vi "Commit DAQ Tags.vi"(8 "error in (no error)":errorcluster, 11 "DAQ State in":T1) -> (0 "error out":errorcluster, 3 "DAQ State out":T1)   [LabVIEW 2018, in "DAQ.lvlib"]
uses:
  DAQ.lvlib
  Acquisition/Hardware Configuration.ctl
  Acquisition/Task Cluster.ctl
  Tag VIs/Tag FGV Operation Enum.ctl
  Shared Variables/Dynamic Shared Variables.lvlib
  <resource>/objmgr/daqmx.rc
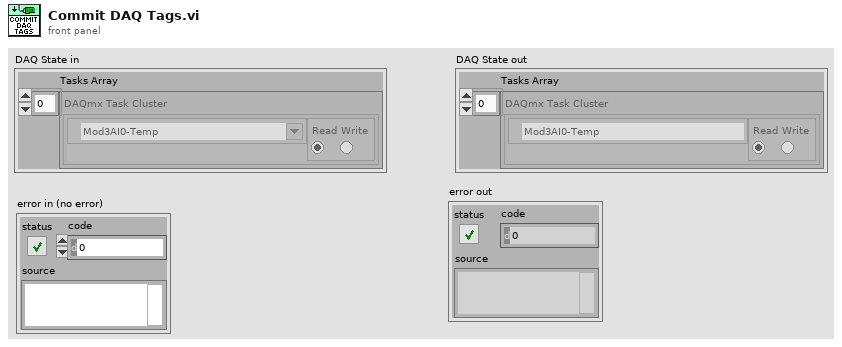
[diagram p1: front panel]
types:
  T1 = typedef "DAQ.lvlib/Hardware Configuration.ctl" = cluster{"Tasks Array":T2[]}
  T2 = typedef "Task Cluster.ctl" = cluster{"DAQmx Task":refnum<k21>, "Read-Write Radio":enum32{"Read", "Write"}}
  T3 = typedef "Tag FGV Operation Enum.ctl" = enum16{"Init", "Set Notification Queue", "Create Tag", "Commit", "Write Tag (Numeric)", "Write Tag (Boolean)", "Read All Tags", "Read One Tag", "Delete Tag Category", "Set Alarm Parameters (Numeric)", "Set Alarm Parameters (Boolean)", "Enable All Alarms", "Disable All Alarms", "Delete All Tags", "Read Alarms", "Ack Alarm", "Read Alarm Parameters (Numeric)", "Read Alarm Parameters (Boolean)"}
  T4 = cluster{"enable? (F)":bool, "name":string, "alarm on":bool, "priority":u32, "ack type":enum16{"Auto", "User", "None", "Each Occurrence"}, "area":string, "description":string, "log? (T)":bool}
  T5 = enum16{"Auto", "User", "None", "Each Occurrence"}
  T6 = enum32{"u32BitField", "bool", "double", "string", "int8", "uint8", "int16", "uint16", "int32", "uint32", "int64", "uint64", "single", "double waveform", "int16 waveform", "array of boolean", "array of int8", "array of uint8", "array of int16", "array of uint16", "array of int32", "array of uint32", "array of int64", "array of uint64", "array of single", "array of double", "array of double waveform", "array of int16 waveform", "array of string", "variant", "timestamp", "fixed point", "custom"}
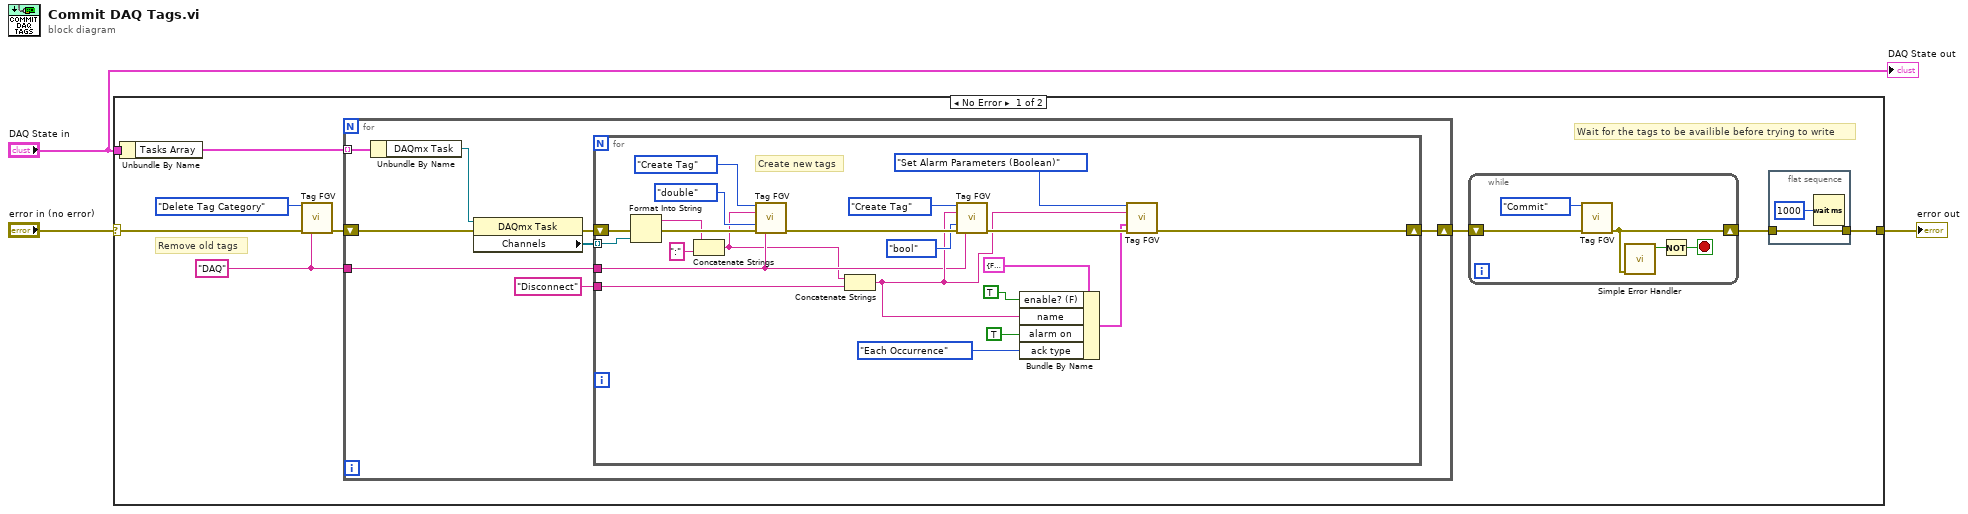
[diagram p0: block diagram]
diagram:
  n1 = case shown="No Error" "error in (no error)" {
    selector: "error in (no error)" -> [w9 w50]
    tunnel: "DAQ State in" -> [w11 _]
    tunnel: [w4 w50] -> w1
    frame No Error {
      w7 = "DAQ" ("Tag Category")
      # "Wait for the tags to be availible before trying to write"
      # "Remove old tags"
      n2 = Unbundle By Name(w11) -> ("Tasks Array"=w12:T2[])
      n3 = call "Tag FGV.vi"("Operation"=Tag_FGV_Operation_Enum."Delete Tag Category", "error in (no error)"=w9, "Tag Category"=w7) -> ("error out"=w8:errorcluster)  [unwired: 5 in, 7 out]
      n4 = for {
        tunnel: w12 -> [w27] mode=indexing
        shift-right: [w22] -> w6
        shift-left: w8 -> [w26]
        tunnel: w7 -> [w23]
        n5 = Unbundle By Name(w27) -> ("DAQmx Task"=w25:refnum<k21>)
        n6 = property class="DAQmx Task"(reference=w25, error in=w26) -> (error out=w21:errorcluster, "Channels"=w24:refnum<k21>[])  [unwired: 1 out]
        n7 = for {
          tunnel: w24 -> [w48] mode=indexing
          shift-right: [w39] -> w22
          shift-left: w21 -> [w47]
          tunnel: w23 -> [w31]
          tunnel: "Disconnect" ("string") -> [w32]
          # "Create new tags"
          n8 = Format Into String(error in=w47, w48) -> (resulting string=w30:string, error out=w49:errorcluster)  [unwired: 2 in]
          n9 = Concatenate Strings(w30, ":" ("string")) -> (w28:string)
          n10 = call "Tag FGV.vi"("Operation"=Tag_FGV_Operation_Enum."Create Tag", "Tag Name"=w28, "Data"=T6."double" ("data type"), "error in (no error)"=w49, "Tag Category"=w31) -> ("error out"=w44:errorcluster)  [unwired: 3 in, 7 out]
          n11 = Concatenate Strings(w28, w32) -> (w36:string)
          n12 = call "Tag FGV.vi"("Operation"=Tag_FGV_Operation_Enum."Create Tag", "Tag Name"=w36, "Data"=T6."bool" ("data type"), "error in (no error)"=w44, "Tag Category"=w31) -> ("error out"=w40:errorcluster)  [unwired: 3 in, 7 out]
          n13 = Bundle By Name(cluster=T4 {"enable? (F)"=FALSE, "name"="Boolean", "alarm on"=TRUE, "priority"=1, "ack type"=enum."Auto", "area"="", "description"="", "log? (T)"=TRUE} ("Boolean alarm settings"), "enable? (F)"=TRUE, "name"=w36, "alarm on"=TRUE, "ack type"=T5."Each Occurrence") -> (w33:T4)
          n14 = call "Tag FGV.vi"("Operation"=Tag_FGV_Operation_Enum."Set Alarm Parameters (Boolean)", "Tag Name"=w36, "Data"=w33, "error in (no error)"=w40) -> ("error out"=w39:errorcluster)  [unwired: 4 in, 7 out]
        }
      }
      n15 = while {
        shift-right: [w17] -> w5
        shift-left: w6 -> [w18]
        stop <- w15 stop-if-true
        n16 = call "Tag FGV.vi"("Operation"=Tag_FGV_Operation_Enum."Commit", "error in (no error)"=w18) -> ("error out"=w17:errorcluster)  [unwired: 6 in, 7 out]
        n17 = call <vilib>:"Simple Error Handler.vi"("error in (no error)"=w17) -> ("error?"=w16:bool)  [unwired: 4 in, 4 out]
        n18 = Not(x=w16) -> (.not. x?=w15:bool)
      }
      n19 = flat-sequence {
        tunnel: [w13] -> w4
        tunnel: w5 -> [w13]
        frame #0 {
          n20 = Wait (ms)(milliseconds to wait=u32 1000) -> ()  [unwired: 1 out]
        }
      }
    }
    frame Error {
    }
  }
  "error out" <- w1
  "DAQ State out" <- "DAQ State in"
